vi "LV to ITX R+coord.vi"(10 "coordinates file path":path, 11 "ibw file path":path=path "C:/Work/IBW - LVArray/BTOCu1005.ibw") -> ()   [LabVIEW 2016, in "LVtoITX.lvclass"]
uses:
  LVtoITX.lvclass
  <vilib>/Utility/file.llb/Read Delimited Spreadsheet (string).vi
  <vilib>/Utility/file.llb/Read Delimited Spreadsheet (DBL).vi
panel:
  in  "Commands":string
  in  "Notes":string
  out "String":string
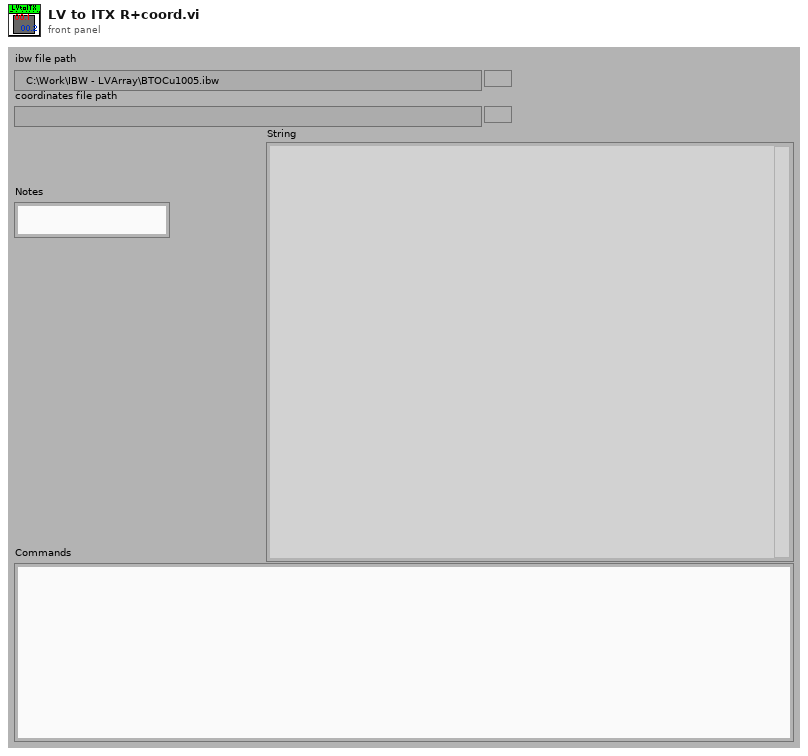
[diagram p1: front panel]
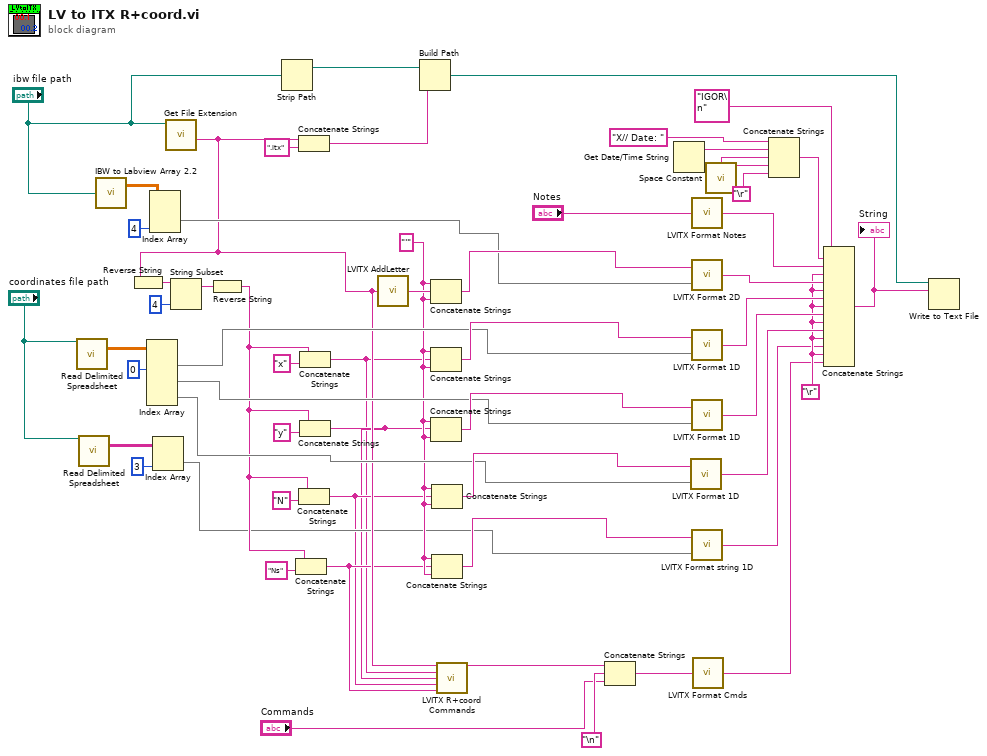
[diagram p0: block diagram]
diagram:
  w18 = "'" ("string")
  w22 = "\r"
  n1 = call-poly <vilib>:"Read Delimited Spreadsheet.vi"("file path (dialog if empty)"="coordinates file path") -> ("all rows"=w33:dbl[][])  [unwired: 9 in, 5 out]
  n2 = call-poly <vilib>:"Read Delimited Spreadsheet.vi"("file path (dialog if empty)"="coordinates file path") -> ("all rows"=w1:string[][])  [unwired: 9 in, 5 out]
  n3 = call <userlib>:"IBW to Labview Array 2.2.vi"("file path (dialog if empty)"="ibw file path") -> ("Output Array"=w36:dbl[][][])  [unwired: 1 out]
  n4 = Index Array(array=w33, index (col) #1=0 ("disabled index (col)")) -> (element #1=w29:dbl[], element #2=w30:dbl[], element #3=w31:dbl[])  [unwired: 5 in]
  n5 = Index Array(array=w36, index (dim 2)=4 ("disabled index (col)")) -> (element=w34:dbl[][])  [unwired: 2 in]
  n6 = Index Array(array=w1, index (col)=3 ("disabled index (col)")) -> (element=w6:string[])  [unwired: 1 in]
  n7 = call <vilib>:"Get File Extension.vi"("file"="ibw file path") -> ("filename without extension"=w12:string)  [unwired: 1 in, 9 out]
  n8 = Reverse String(1:w12) -> (0:w11:string)
  n9 = String Subset(string=w11, length (rest)=4 ("length (rest)")) -> (substring=w10:string)  [unwired: 1 out]
  n10 = Reverse String(1:w10) -> (0:w9:string)
  n11 = Strip Path(path="ibw file path") -> (stripped path=w15:path)  [unwired: 1 out]
  n12 = Concatenate Strings(w9, "Ns" ("string")) -> (w5:string)
  n13 = Concatenate Strings(w12, ".itx" ("string")) -> (w14:string)
  n14 = Concatenate Strings(w9, "N" ("string")) -> (w4:string)
  n15 = Concatenate Strings(w9, "x" ("string")) -> (w2:string)
  n16 = Concatenate Strings(w9, "y" ("string")) -> (w3:string)
  n17 = call "LVITX AddLetter.vi"("String"=w12) -> ("output string"=w42:string)
  n18 = Build Path(base path=w15, name or relative path=w14) -> (appended path=w13:path)
  n19 = Concatenate Strings(w18, w42, w18) -> (w39:string)
  n20 = Concatenate Strings(w18, w2, w18) -> (w40:string)
  n21 = Concatenate Strings(w18, w3, w18) -> (w41:string)
  n22 = Concatenate Strings(w18, w4, w18) -> (w37:string)
  n23 = Concatenate Strings(w18, w5, w18) -> (w19:string)
  n24 = call "LVITX R+coord Commands.vi"("2D wavename"=w12, "X wavename"=w2, "Y wavename"=w3, "N wavename"=w4, "Ns wavename"=w5) -> ("result string"=w38:string)  [unwired: 1 in, 9 out]
  n25 = Concatenate Strings(w38, "\n", "Commands") -> (w45:string)
  n26 = Get Date/Time String() -> (date string=w57:string, time string=w58:string)  [unwired: 3 out]
  n27 = call "LVITX Format 1D.vi"("X 1D Array"=w31, "X  Array name"=w37) -> ("String"=w23:string)
  n28 = call "LVITX Format Notes.vi"("Notes"="Notes") -> ("String"=w49:string)
  n29 = call "LVITX Format 2D.vi"("2D Array"=w34, "2D Array name"=w39) -> ("String"=w52:string)
  n30 = call "LVITX Format 1D.vi"("X 1D Array"=w29, "X  Array name"=w40) -> ("String"=w51:string)
  n31 = call "LVITX Format 1D.vi"("X 1D Array"=w30, "X  Array name"=w41) -> ("String"=w50:string)
  n32 = call "LVITX Format string 1D.vi"("X 1D Array"=w6, "X  Array name"=w19) -> ("String"=w20:string)
  n33 = call "LVITX Format Cmds.vi"("Commands"=w45) -> ("String"=w21:string)
  n34 = call <vilib>:"Space Constant.vi"() -> ("String"=w47:string)
  n35 = Concatenate Strings("X// Date: " ("format string"), w57, w47, w58, "\r") -> (w56:string)
  n36 = Concatenate Strings("IGOR\n", w56, w49, w22, w52, w22, w51, w22, w50, w22, w23, w22, w20, w22, w21) -> (w48:string)
  "String" <- w48
  n37 = Write to Text File(file (use dialog)=w13, text=w48) -> ()  [unwired: 1 in, 4 out]
